vi "sub vi-open serial port v1.vi"(0 "Select COM port":refnum<visa-resource-name>) -> (4 "Error":bool, 6 "LOOPS":i32, 8 "VISA Com out":refnum<visa-resource-name>)   [LabVIEW 2017]
uses:
  <vilib>/Instr/_visa.llb/VISA Configure Serial Port (Instr).vi
panel:
  # "BUSY CONFIGURING SERIAL PORT"
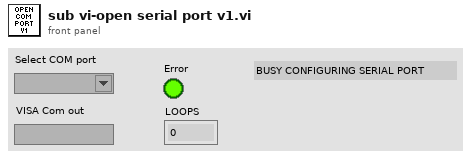
[diagram p1: front panel]
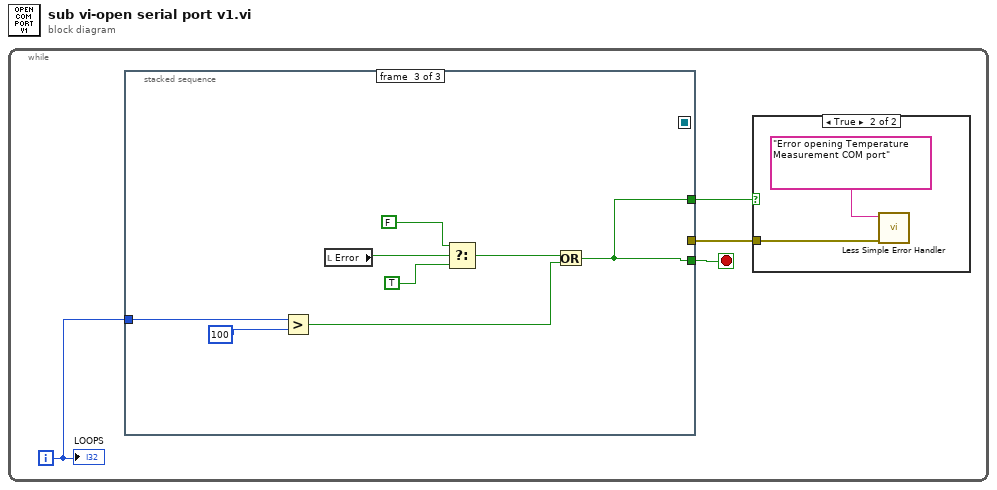
[diagram p0: block diagram]
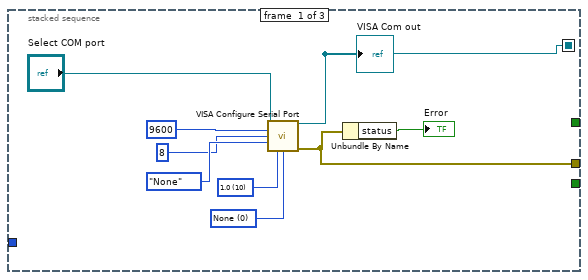
[diagram p3: hidden frame]
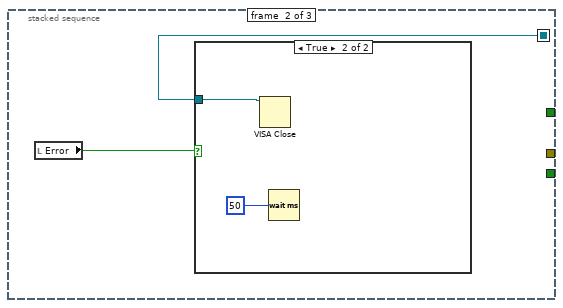
[diagram p4: hidden frame]
diagram:
  n1 = while {
    i -> [w3]
    stop <- w4 stop-if-true
    n2 = stacked-sequence {
      seq-local: [w8 _ _] -> [_ w16 _]
      tunnel: [_ _ w20] -> w4
      tunnel: w3 -> [_ _ w25]
      tunnel: [_ _ w20] -> w2
      tunnel: [w7 _ _] -> w1
      frame #0 {
        w14 = u16 0 items=["None", "XON/XOFF", "RTS/CTS", "XON/XOFF & RTS/CTS", "DTR/DSR", "XON/XOFF & DTR/DSR"] ("flow control (0:none)")
        w13 = u16 10 items=["1.0"=10, "1.5"=15, "2.0"=20] ("stop bits (10: 1 bit)")
        n3 = call-poly "VISA Configure Serial Port"("VISA resource name"="Select COM port", "baud rate (9600)"=u32 9600, "data bits (8)"=u16 8, "parity (0:none)"=enum16{"None", "Odd", "Even", "Mark", "Space"}."None", "stop bits (10: 1 bit)"=w13, "flow control (0:none)"=w14) -> ("VISA resource name out"=w8:refnum<visa-resource-name>, "error out"=w7:errorcluster)  [unwired: 8 in]
        "VISA Com out" <- w8
        n4 = Unbundle By Name(w7) -> ("status"=→"Error":bool)
      }
      frame #1 {
        n5 = local read "Error"() -> (w17:bool)
        n6 = case shown="True" w17 {
          tunnel: w16 -> [_ w18]
          frame False {
          }
          frame True {
            n7 = VISA Close(VISA resource name=w18) -> ()  [unwired: 1 in, 1 out]
            n8 = Wait (ms)(milliseconds to wait=50) -> ()  [unwired: 1 out]
          }
        }
      }
      frame #2 {
        n9 = Greater?(x=w25, y=100) -> (0:w23:bool)
        n10 = local read "Error"() -> (w27:bool)
        n11 = Select(t=FALSE, s=w27, f=TRUE) -> (s? t:f=w21:bool)
        n12 = Or(x=w21, y=w23) -> (x .or. y?=w20:bool)
      }
    }
    n13 = case shown="True" w2 {
      tunnel: w1 -> [_ w5]
      frame False {
      }
      frame True {
        n14 = call "Less Simple Error Handler.vi"("message"="Error opening Temperature Measurement COM port", "error in"=w5) -> ()  [unwired: 4 in]
      }
    }
    "LOOPS" <- w3
  }
